vi "Global 1.vi"() -> ()   [LabVIEW 2021]
panel:
  in  "appended array":cluster{"Ramp Pattern":dbl[], u32[]}[](array[cluster])
  in  "Curva de luz cruda":cluster{"Ramp Pattern":dbl[], u32[]}(graph)
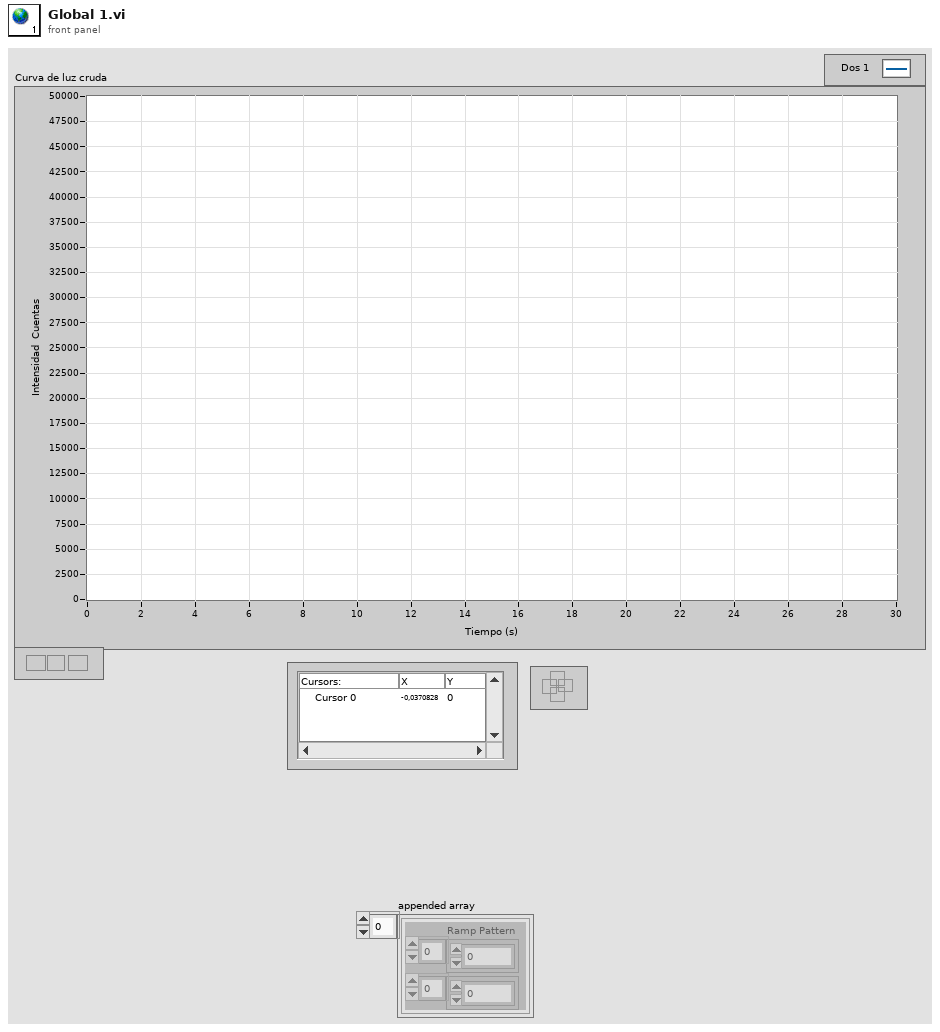
[diagram p1: front panel]
diagram:
